vi "Set SubPanel.vi"(8 "error in (no error)":errorcluster, 10 "SubPanel":refnum<vi>, 11 "Brower View in":refnum<class "Brower View.lvclass">) -> (0 "error out":errorcluster, 3 "Brower View out":refnum<class "Brower View.lvclass">)   [LabVIEW 2015, in "Brower View.lvclass"]
uses:
  Brower View.lvclass
  Brower View.lvclass/Brower View.ctl
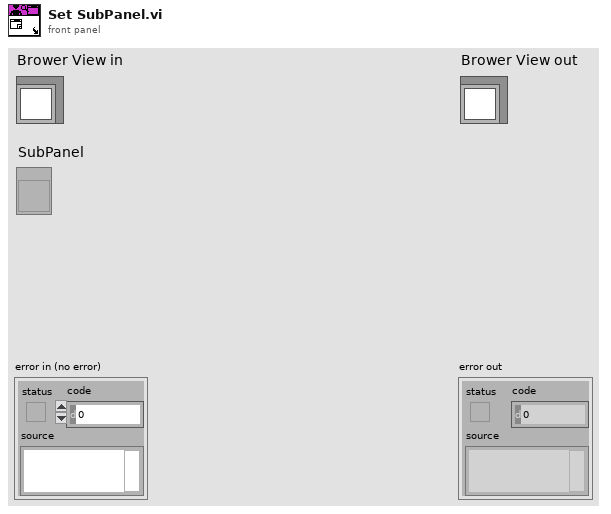
[diagram p1: front panel]
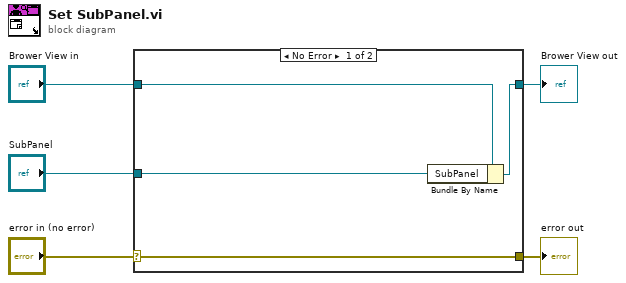
[diagram p0: block diagram]
diagram:
  n1 = case shown="No Error" "error in (no error)" {
    selector: "error in (no error)" -> [w9 w10]
    tunnel: [w9 w10] -> w4
    tunnel: [w7 w11] -> w2
    tunnel: "Brower View in" -> [w8 w11]
    tunnel: "SubPanel" -> [w6 _]
    frame No Error {
      n2 = Bundle By Name(cluster=w8, "SubPanel"=w6) -> (w7:refnum<class "Brower View.lvclass">)
    }
    frame Error {
    }
  }
  "error out" <- w4
  "Brower View out" <- w2
